vi "getVolumeDescriptor.vi"(8 "error in (no error)":errorcluster, 11 "VGS_Project in":refnum<class "VGS_Project.lvclass">) -> (0 "error out":errorcluster, 2 "VGS_VolumeDescriptor out":refnum<class "VGS_VolumeDescriptor.lvclass">, 3 "VGS_Project out":refnum<class "VGS_Project.lvclass">)   [LabVIEW 2022 SP3, in "LV_VGS.lvlib" / "VGS_Project.lvclass"]
uses:
  VGS_Project.lvclass
  VolumeDescriptor/VGS_VolumeDescriptor.lvclass
  VGS_Project.lvclass/VGS_Project.ctl
  C:/Users/Andrey/Desktop/hajo/LV_VGS/vgs_project.dll
  vgs_project.dll
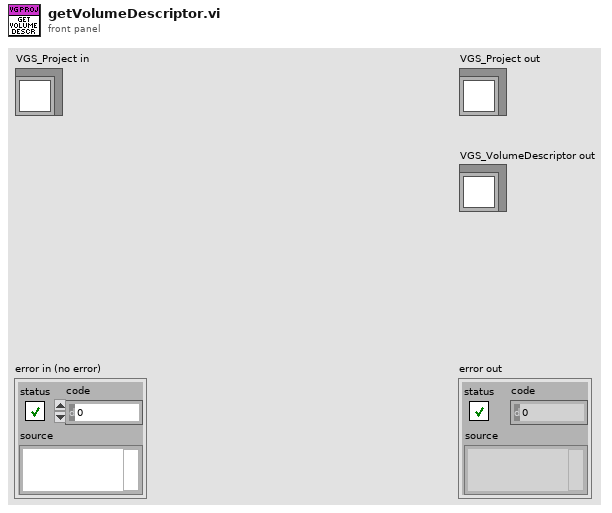
[diagram p1: front panel]
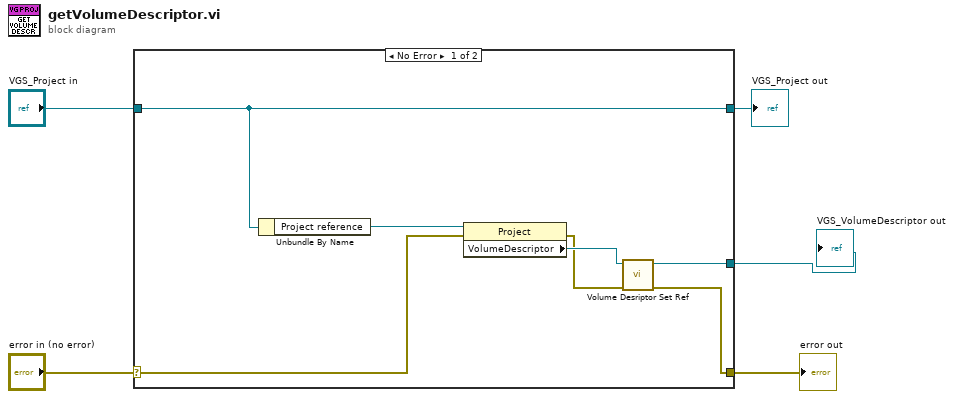
[diagram p0: block diagram]
diagram:
  n1 = case shown="No Error" "error in (no error)" {
    selector: "error in (no error)" -> [w10 w14]
    tunnel: [w6 w14] -> w1
    tunnel: [w12 w13] -> w3
    tunnel: "VGS_Project in" -> [w12 w13]
    tunnel: [w8 _] -> w2
    frame No Error {
      n2 = Unbundle By Name(w12) -> ("Project reference"=w11:refnum<k24>)
      n3 = property class="Project"(reference=w11, error in=w10) -> (error out=w7:errorcluster, "VolumeDescriptor"=w9:refnum<k24>)  [unwired: 1 out]
      n4 = call "Volume Desriptor Set Ref.vi"("error in (no error)"=w7, "VolumeDescriptor"=w9) -> ("error out"=w6:errorcluster, "VGS_VolumeDescriptor out"=w8:refnum<class "VGS_VolumeDescriptor.lvclass">)  [unwired: 8 in]
    }
    frame Error {
    }
  }
  "error out" <- w1
  "VGS_Project out" <- w3
  "VGS_VolumeDescriptor out" <- w2
